vi "Tree_Tag Delimiter.vi"() -> (3 "Tree Tag delimiter":string)   [LabVIEW 2023]
doc: "Tree heirarchy is carried in a string with a delimiter that is a combination of characters unlikely to ever be found in a contol lablel.\n\nWe could check every control lable for this delimiter and create a new one on the fly if needed, but this will probably work.\n\nBefore, I was using a dot delimiter, but this didn't work with controls with dots in their names."
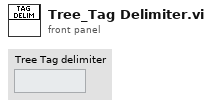
[diagram p1: front panel]
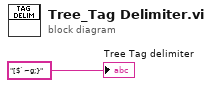
[diagram p0: block diagram]
diagram:
  "Tree Tag delimiter" <- "[$`~g;}" ("Tree Tag delimiter")
